vi "Initialize_NI.vi"(0 "Motion Settings":T2={"No Motion?"=FALSE, "Motion System"=enum."NI 735x", "Motion Bd ID"=1, "Motion Profile"="SMAC1", "# Axis"=1, "Reverse Z axis?"=TRUE, "SMAC Axis"=0, "scan pair"=enum."y-(x) scan", "RT fps"=6.0, "Steps per mm"=[1000, 1000, 1000, 1000], "Motor Parameters"={"velocity ct/s"=[10000.0, 10000.0, 10000.0, 50000.0], "accel ct/s^2"=[50000.0, 50000.0, 50000.0, 200000.0]}, "One Way Scan"=FALSE, "Reverse One Way Scan"=FALSE, "Global Position (mm)"=[], "Plane"=0, "Distance between\nscan lines (um)"=0.0, "Distance between\nscan planes (um)"=0.0, "number of scan planes"=1, "Total steps in line"=0, "Xtra plane\ndistance  (um)"=100, "Xtra planes "=1, "Add Axis"=FALSE, "overshoot cts"=200, "BKPT Shift"=0, "Scan Start Time (ms)"=0, "ESP VISA"="GPIB::1::INSTR", "3rd Axis"=1, "GL Ref Out"=refnum, "Galil Address"=""} {"3rd Axis" items=["x", "y", "z", "w"]; "Xtra planes" min=1; "Xtra plane\ndistance  (um)" min=0; "Distance between\nscan planes (um)" format="%.2f"; "Distance between\nscan lines (um)" format="%.2f"; "SMAC Axis" items=["None"=0, "Axis 1"=1, "Axis 2"=2, "Axis 3"=3, "Axis 4"=4, "Axis 5"=5, "Axis 6"=6, "Axis 7"=7, "Axis 8"=8, "Vector Space 1"=17, "Vector Space 2"=18, "Vector Space 3"=19, "Vector Space 4"=20]; "Motion Bd ID" min=1 max=32 step=1}, 1 "Bypass Motion Init":bool, 2 "Location":T1, 3 "error in":errorcluster) -> (5 "Bd ID Out":u8, 6 "Initialization Failed!!":bool, 7 "error out":errorcluster)   [LabVIEW 2022 SP3]
uses:
  MotionParameters.ctl
  MotionSys.ctl
  -MotionRoutines/ScanAxis.ctl
  -MotionRoutines/3rdAxis.ctl
  -ScanSystem/Controls/location.ctl
  <vilib>/Motion/FlexMotion/FunctionsVIs/Trajectory.llb/Load Acceleration/Deceleration.flx
  <vilib>/Motion/FlexMotion/CustomControls/CustomControls.llb/Mask (8 axes).flx
  <vilib>/Motion/FlexMotion/CustomControls/CustomControls.llb/Axis To Configure.flx
  <vilib>/Motion/FlexMotion/CustomControls/CustomControls.llb/ControlGainParameter.flx
  <vilib>/Motion/FlexMotion/FunctionsVIs/MotionIO.llb/Set Breakpoint Output MOMO (8 axes).flx
panel:
  # "1-D and 2-D B scan settings"
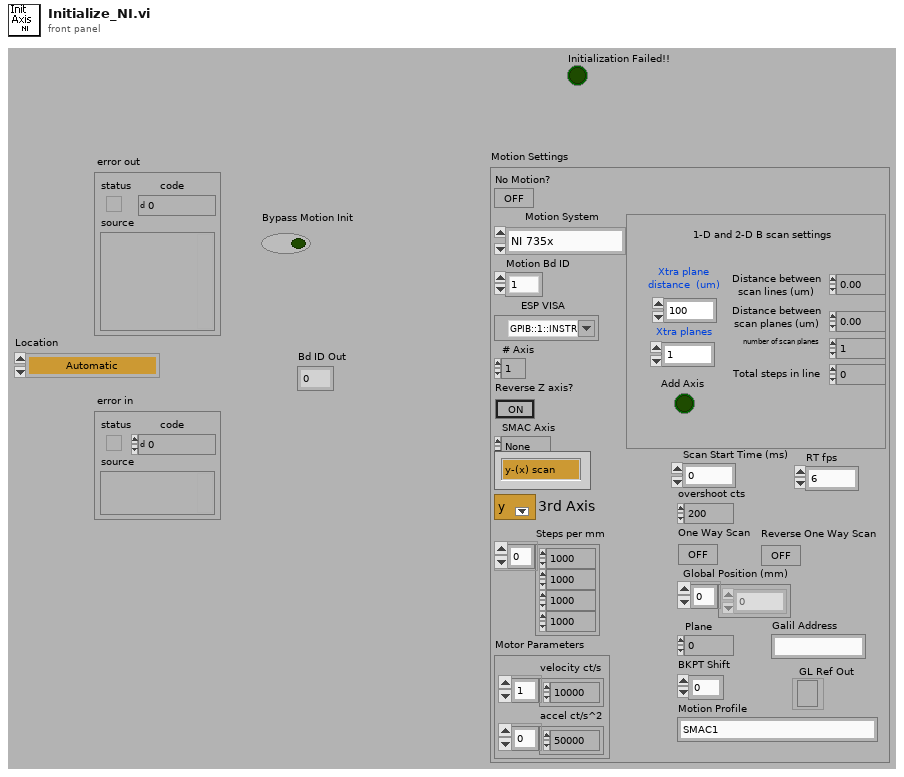
[diagram p1: front panel]
types:
  T1 = typedef "location.ctl" = enum16{"Automatic", "WCM Main", "Hawaii", "Columbia MM3000", "Columbia  NI System", "NYU", "RRI 2", "UHI Allen", "CUMC RT", "Chiba", "Stony Brook", "WCM Microscopy", "WCM Aeoretch", "WCM Optics Lab", "WCM Main 2Axis", "WCM Rotation", "WCM SAM SMAC", "SERI GP"}
  T2 = typedef "MotionParameters.ctl" = cluster{"No Motion?":bool, "Motion System":T3, "Motion Bd ID":u8, "Motion Profile":string, "# Axis":i8, "Reverse Z axis?":bool, "SMAC Axis":u16, "scan pair":T4, "RT fps":sgl, "Steps per mm":i32[], "Motor Parameters":cluster{"velocity ct/s":dbl[], "accel ct/s^2":dbl[]}, "One Way Scan":bool, "Reverse One Way Scan":bool, "Global Position (mm)":dbl[], "Plane":i32, "Distance between\nscan lines (um)":sgl, "Distance between\nscan planes (um)":sgl, "number of scan planes":i32, "Total steps in line":i32, "Xtra plane\ndistance  (um)":i32, "Xtra planes ":i32, "Add Axis":bool, "overshoot cts":i32, "BKPT Shift":i32, "Scan Start Time (ms)":u32, "ESP VISA":refnum<visa-resource-name>, "3rd Axis":T5, "GL Ref Out":refnum<k7>, "Galil Address":string}
  T3 = typedef "MotionSys.ctl" = enum16{"MM3000", "NI 735x", "Newport ESP", "No Motion Card", "Galil"}
  T4 = typedef "ScanAxis.ctl" = enum16{"y-(x) scan", "x-(y) scan", "z-(x) scan", "z-(y) scan", "y-(z) scan", "x-(z) scan", "w-(x) scan", "w-(y) scan", "w-(z) scan", "x-(w) scan", "y-(w) scan", "z-(w) scan"}
  T5 = typedef "3rdAxis.ctl" = u16
  T6 = typedef "ControlGainParameter.flx" = enum16{"Kp", "Ki", "IL", "Kd", "Td", "Kv", "Aff", "Vff"}
  T7 = typedef "Mask (8 axes).flx" = cluster{"1":bool, "2":bool, "3":bool, "4":bool, "5":bool, "6":bool, "7":bool, "8":bool}
  T8 = enum16{"Left Button", "Center Button", "Right Button", "Window Close"}
  T9 = typedef "Axis To Configure.flx" = u16
  T10 = typedef "Bd Id Out" = u8
  T11 = typedef "Axis Status (8 axes).flx" = cluster{"1":bool, "2":bool, "3":bool, "4":bool, "5":bool, "6":bool, "7":bool, "8":bool}
  T12 = typedef "Resource Out (Enum).flx" = u16
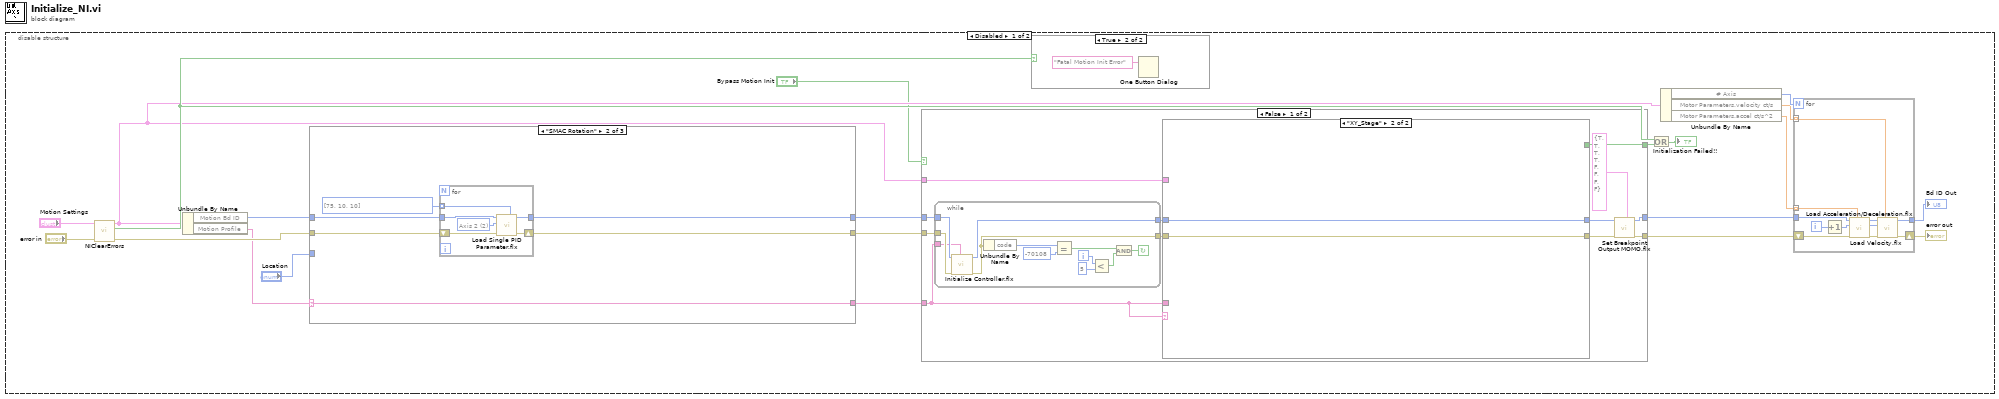
[diagram p0: block diagram]
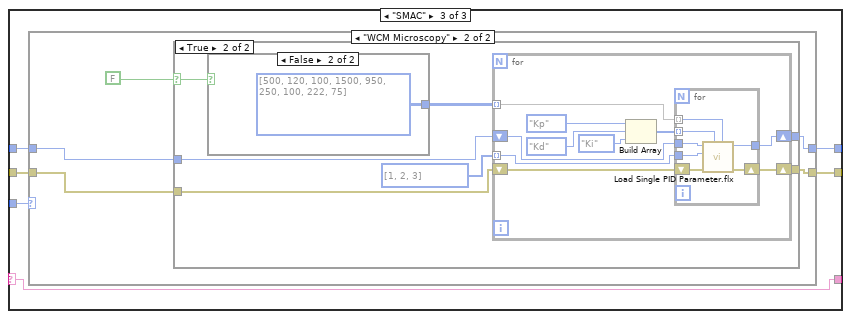
[diagram p4: hidden frame]
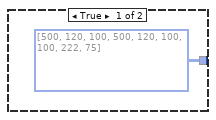
[diagram p7: hidden frame]
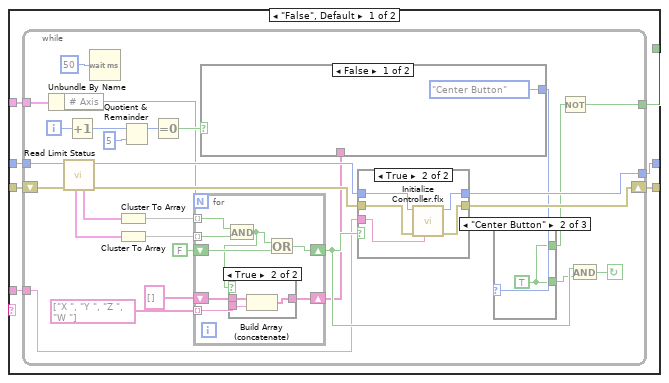
[diagram p8: hidden frame]
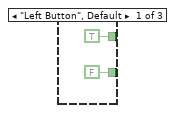
[diagram p9: hidden frame]
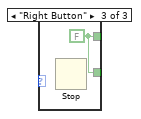
[diagram p10: hidden frame]
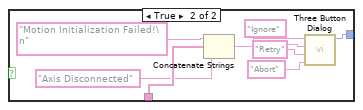
[diagram p12: hidden frame]
diagram:
  n1 = disable-structure shown="Disabled" {
    frame Disabled {
      n2 = call "NIClearErrors.vi"("error in (no error)"="error in", "Motion Settings"="Motion Settings") -> ("error out"=w12:errorcluster, "Error?"=w6:bool, "Motion Settings Out"=w3:T2)  [unwired: 7 in]
      n3 = Unbundle By Name(w3) -> ("Motion Bd ID"=w5:u8, "Motion Profile"=w1:string)
      n4 = case shown="\"SMAC Rotation\"" w1 {
        selector: w1 -> [w23 w26 w39]
        tunnel: w5 -> [w25 w31 w43]
        tunnel: [w25 w28 w41] -> w13
        tunnel: w12 -> [w24 w29 w42]
        tunnel: [w24 w27 w40] -> w11
        tunnel: [w23 w26 w39] -> w10
        tunnel: "Location" -> [_ _ w38]
        frame "False", Default {
        }
        frame "SMAC Rotation" {
          n5 = for {
            tunnel: w31 -> [w37]
            tunnel: [w36] -> w28
            tunnel: i32[] [75, 10, 10] -> [w34] mode=indexing
            shift-right: [w33] -> w27
            shift-left: w29 -> [w32]
            w35 = T9 2 items=["Axis 1"=1, "Axis 2"=2, "Axis 3"=3, "Axis 4"=4, "Axis 5"=5, "Axis 6"=6, "Axis 7"=7, "Axis 8"=8] ("Axis")
            n6 = call <vilib>:"Load Single PID Parameter.flx"("Value (0)"=w34, "error in (no error)"=w32, "Axis"=w35, "Board ID"=w37) -> ("error out"=w33:errorcluster, "Bd ID Out"=w36:T10)  [unwired: 3 in, 1 out]
          }
        }
        frame "SMAC" {
          n7 = case shown="\"WCM Microscopy\"" w38 {
            tunnel: w43 -> [w44 w50]
            tunnel: w42 -> [w45 w49]
            tunnel: [w44 w48] -> w41
            tunnel: [w45 w47] -> w40
            frame "Automatic", Default {
            }
            frame "WCM Microscopy" {
              n8 = case shown="True" FALSE {
                selector: FALSE -> [_ w53]
                tunnel: w50 -> [w52 w59]
                tunnel: w49 -> [w51 w57]
                tunnel: [w52 w56] -> w48
                tunnel: [w51 w55] -> w47
                frame False {
                }
                frame True {
                  w54 = T9[] [1, 2, 3] items=["Axis 1"=1, "Axis 2"=2, "Axis 3"=3, "Axis 4"=4, "Axis 5"=5, "Axis 6"=6, "Axis 7"=7, "Axis 8"=8] ("Array")
                  n9 = case shown="False" w53 {
                    tunnel: [i32[][] [[500, 120, 100], [500, 120, 100], [100, 222, 75]] i32[][] [[500, 120, 100], [1500, 950, 250], [100, 222, 75]]] -> w58
                    frame True {
                    }
                    frame False {
                    }
                  }
                  n10 = for {
                    tunnel: w58 -> [w70] mode=indexing
                    tunnel: w54 -> [w66] mode=indexing
                    shift-right: [w68] -> w56
                    shift-left: w59 -> [w71]
                    shift-right: [w67] -> w55
                    shift-left: w57 -> [w69]
                    n11 = Build Array(ControlGainParameter.flx."Kp" ("Parameter (Kp)"), ControlGainParameter.flx."Kd" ("Parameter (Kp)"), ControlGainParameter.flx."Ki" ("Parameter (Kp)")) -> (w63:T6[])
                    n12 = for {
                      tunnel: w71 -> [w78]
                      tunnel: [w77] -> w68
                      tunnel: w70 -> [w76] mode=indexing
                      shift-right: [w75] -> w67
                      shift-left: w69 -> [w74]
                      tunnel: w66 -> [w73]
                      tunnel: w63 -> [w72] mode=indexing
                      n13 = call <vilib>:"Load Single PID Parameter.flx"("Value (0)"=w76, "Parameter (Kp)"=w72, "error in (no error)"=w74, "Axis"=w73, "Board ID"=w78) -> ("error out"=w75:errorcluster, "Bd ID Out"=w77:T10)  [unwired: 2 in, 1 out]
                    }
                  }
                }
              }
            }
          }
        }
      }
      n14 = case shown="False" "Bypass Motion Init" {
        tunnel: w13 -> [w101 w185]
        tunnel: w10 -> [w90 _]
        tunnel: [w98 w185] -> w17
        tunnel: [w97 w184] -> w16
        tunnel: w11 -> [w100 w184]
        tunnel: [w91 _] -> w7
        tunnel: w3 -> [w94 _]
        frame False {
          n15 = while {
            tunnel: w101 -> [w183]
            tunnel: w90 -> [w181]
            tunnel: [w180] -> w92
            tunnel: w100 -> [w182]
            tunnel: [w179] -> w93
            i -> [w174]
            stop <- w176 continue-if-true
            n16 = call <vilib>:"Initialize Controller.flx"("Settings Name"=w181, "error in (no error)"=w182, "Board ID"=w183) -> ("error out"=w179:errorcluster, "Bd ID Out"=w180:T10)  [unwired: 5 out]
            n17 = Unbundle By Name(w179) -> ("code"=w178:i32)
            n18 = Equal?(x=w178, y=-70108) -> (x = y?=w175:bool)
            n19 = Less?(x=w174, y=5) -> (x < y?=w172:bool)
            n20 = And(x=w175, y=w172) -> (x .and. y?=w176:bool)
          }
          n21 = case shown="\"XY_Stage\"" w90 {
            tunnel: w90 -> [w108 _]
            tunnel: [w107 w171] -> w96
            tunnel: [w106 w170] -> w95
            tunnel: w94 -> [w105 _]
            tunnel: w93 -> [w104 w170]
            tunnel: w92 -> [w103 w171]
            tunnel: [w102 _] -> w91
            frame "False", Default {
              n22 = while {
                tunnel: w103 -> [w136]
                tunnel: [w129] -> w107
                shift-right: [w121] -> w106
                shift-left: w104 -> [w137]
                tunnel: w108 -> [w116]
                tunnel: [w122] -> w102
                tunnel: w105 -> [w117]
                i -> [w126]
                stop <- w123 continue-if-true
                n23 = Unbundle By Name(w117) -> ("# Axis"=w115:i8)
                n24 = call <vilib>:"Read Limit Status.vi"("error in (no error)"=w137, "Board ID"=w136) -> ("error out"=w120:errorcluster, "Bd ID Out"=w130:T10, "Reverse Limits"=w135:T11, "Forward Limits"=w134:T11)  [unwired: 6 in]
                n25 = Increment(x=w126) -> (x+1=w124:i32)
                n26 = Wait (ms)(milliseconds to wait=u32 50) -> ()  [unwired: 1 out]
                n27 = Cluster To Array(cluster=w135) -> (array=w133:bool[])
                n28 = Cluster To Array(cluster=w134) -> (array=w132:bool[])
                n29 = Quotient & Remainder(x=w124, y=5 ("x")) -> (x-y*floor(x/y)=w127:i32)  [unwired: 1 out]
                n30 = Equal To 0?(x=w127) -> (x = 0?=w128:bool)
                n31 = for {
                  N: w115 -> [_]
                  tunnel: w133 -> [w165] mode=indexing
                  tunnel: w132 -> [w164] mode=indexing
                  shift-right: [w162] -> w119
                  shift-left: FALSE -> [w163]
                  shift-right: [w160] -> w113
                  shift-left: string[] [] -> [w159]
                  tunnel: string[] ["X ", "Y ", "Z ", "W "] -> [w158] mode=indexing
                  n32 = And(x=w165, y=w164) -> (x .and. y?=w161:bool)
                  n33 = case shown="True" w161 {
                    tunnel: [w166 w168] -> w160
                    tunnel: w159 -> [w166 w169]
                    tunnel: w158 -> [_ w167]
                    frame False {
                    }
                    frame True {
                      n34 = Build Array (concatenate)(w169, w167) -> (w168:string[])
                    }
                  }
                  n35 = Or(x=w161, y=w163) -> (x .or. y?=w162:bool)
                }
                n36 = case shown="False" w128 {
                  tunnel: w113 -> [_ w154]
                  tunnel: [T8."Center Button" ("Which Button?") w152] -> w111
                  frame False {
                  }
                  frame True {
                    n37 = Concatenate Strings("Motion Initialization Failed!\n" ("message"), w154, "Axis Disconnected" ("string")) -> (w155:string)
                    n38 = call <vilib>:"Three Button Dialog.vi"("Right Button Text (\"Cancel\")"="Abort" ("F button name (\"Cancel\")"), "Center Button Text (\"No\")"="Retry" ("T button name (\"OK\")"), "Left Button Text (\"Yes\")"="Ignore" ("Right Button Text (\"Cancel\")"), "message"=w155) -> ("Which Button?"=w152:T8)  [unwired: 7 in]
                  }
                }
                n39 = case shown="True" w119 {
                  tunnel: w130 -> [w143 w148]
                  tunnel: [w143 w147] -> w129
                  tunnel: w116 -> [_ w146]
                  tunnel: w120 -> [w142 w145]
                  tunnel: [w142 w144] -> w121
                  frame False {
                  }
                  frame True {
                    n40 = call <vilib>:"Initialize Controller.flx"("Settings Name"=w146, "error in (no error)"=w145, "Board ID"=w148) -> ("error out"=w144:errorcluster, "Bd ID Out"=w147:T10)  [unwired: 5 out]
                  }
                }
                n41 = case shown="\"Center Button\"" w111 {
                  tunnel: [FALSE w140 w141] -> w110
                  tunnel: [TRUE w140 w141] -> w109
                  frame "Left Button", Default {
                  }
                  frame "Center Button" {
                    w140 = TRUE
                  }
                  frame "Right Button" {
                    w141 = FALSE
                    n42 = Stop() -> ()  [unwired: 1 in]
                  }
                }
                n43 = Not(x=w109) -> (.not. x?=w122:bool)
                n44 = And(x=w119, y=w110) -> (x .and. y?=w123:bool)
              }
            }
            frame "XY_Stage" {
            }
          }
          n45 = call-poly <vilib>:"Set Breakpoint Output MOMO.flx"("Must Off (False)"=T7 {"1"=TRUE, "2"=TRUE, "3"=TRUE, "4"=TRUE, "5"=FALSE, "6"=FALSE, "7"=FALSE, "8"=FALSE}, "error in (no error)"=w95, "Board ID"=w96) -> ("error out"=w97:errorcluster, "Bd ID Out"=w98:T10)  [unwired: 3 in, 2 out]
        }
        frame True {
        }
      }
      n46 = case shown="True" w6 {
        frame False {
        }
        frame True {
          n47 = One Button Dialog(message="Fatal Motion Init Error") -> ()  [unwired: 1 in, 1 out]
        }
      }
      n48 = Or(x=w6, y=w7) -> (x .or. y?=→"Initialization Failed!!":bool)
      n49 = Unbundle By Name(w3) -> ("# Axis"=w20:i8, "Motor Parameters.velocity ct/s"=w19:dbl[], "Motor Parameters.accel ct/s^2"=w18:dbl[])
      n50 = for {
        N: w20 -> [_]
        tunnel: w17 -> [w83]
        tunnel: [w88] -> w14
        shift-right: [w87] -> w15
        shift-left: w16 -> [w85]
        tunnel: w19 -> [w86] mode=indexing
        tunnel: w18 -> [w80] mode=indexing
        i -> [w89]
        n51 = Increment(x=w89) -> (x+1=w81:i32)
        n52 = call "Load Acceleration/Deceleration.flx"("Acceleration (100000)"=w80, "error in (no error)"=w85, "Axis or Vector Space"=w81, "Board ID"=w83) -> ("error out"=w84:errorcluster, "Resource Output"=w79:T12, "Bd ID Out"=w82:T10)  [unwired: 1 in, 2 out]
        n53 = call <vilib>:"Load Velocity.flx"("Velocity (10000)"=w86, "error in (no error)"=w84, "Axis or Vector Space"=w79, "Board ID"=w82) -> ("error out"=w87:errorcluster, "Bd ID Out"=w88:T10)  [unwired: 4 out]
      }
      "error out" <- w15
      "Bd ID Out" <- w14
    }
    frame Enabled {
    }
  }
